vi "Filter wheel settings globals.vi"() -> ()   [LabVIEW 2016]
panel:
  in  "Minimum time to wait after filter change (ms)":u32=50
  in  "Filter wheel successful initialization?":bool
  in  "Filter wheel present?":bool=TRUE
  in  "Filter wheel computer port":refnum<visa-resource-name>="FILTERWHEEL"
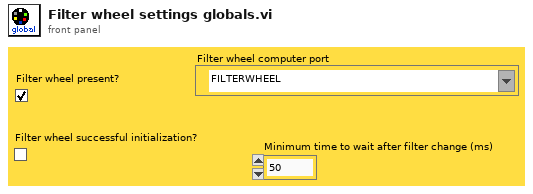
[diagram p1: front panel]
diagram:
